vi "Insert Front Panel.vi"(8 "error in (no error)":errorcluster, 9 "Insertion Request Time":timestamp, 10 "Protected Subpanel":T1, 11 "User Manager View in":refnum<class "User Manager View.lvclass">) -> (0 "error out":errorcluster, 3 "User Manager View out":refnum<class "User Manager View.lvclass">)   [LabVIEW 2017, in "User Manager View.lvlib" / "User Manager View.lvclass"]
doc: "<License>\nCopyright © 2017 Composed Systems, LLC | All rights reserved\nwww.composed.io\n\nAuthor: Ethan Stern <ethan.stern@composed.io>\n\nThis software is provided \"AS IS\" WITHOUT WARRANTIES, either express or implied, AND IS FOR EDUCATIONAL PURPOSES ONLY.\n</License>"
uses:
  User Manager View.lvclass
  <vilib>/gpm_packages/@cs/mva-viewable/Source/IViewable/ProtectedSubpanel/Protected Subpanel Reference.ctl
  <vilib>/gpm_packages/@cs/mva-viewable/Source/IViewable/ProtectedSubpanel/ProtectedSubpanel.lvclass
  User Manager View.lvclass/User Manager View.ctl
  <vilib>/gpm_packages/@cs/mva-viewable/Source/IViewable/IViewable/IViewable.lvclass
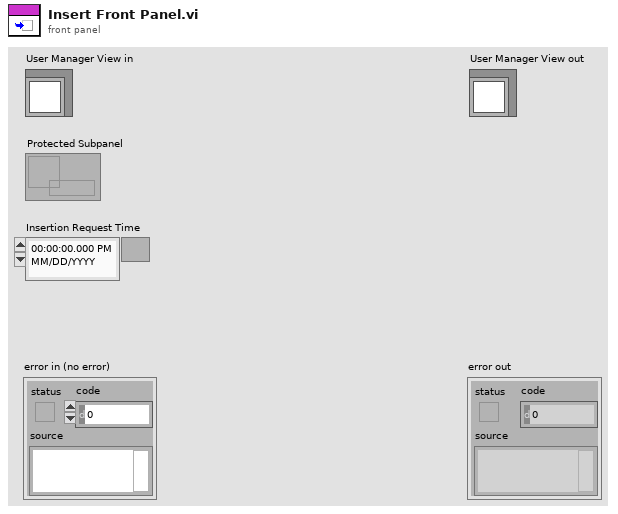
[diagram p1: front panel]
types:
  T1 = typedef "IViewable.lvlib/ProtectedSubpanel.lvclass/Protected Subpanel Reference.ctl" = refnum<data-value>
  T2 = enum8{"Enabled", "Disabled", "Disabled and Grayed Out"}
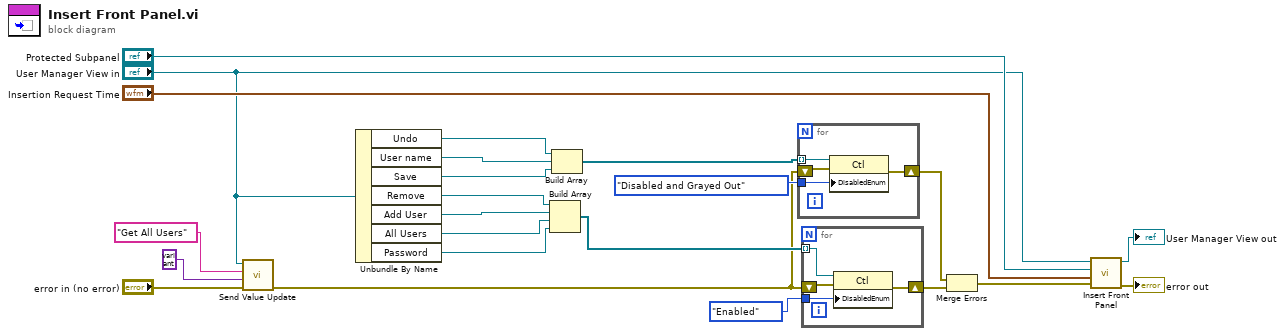
[diagram p0: block diagram]
diagram:
  n1 = call-dynamic "Send Value Update.vi"("error in (no error)"="error in (no error)", "Value"=variant, "Datum Name"="Get All Users", "IViewable in"="User Manager View in") -> ("error out"=w3:errorcluster)  [unwired: 7 in]
  n2 = Unbundle By Name("User Manager View in") -> ("Undo"=w5:refnum<vi>, "User name"=w10:refnum<vi>, "Save"=w9:refnum<vi>, "Remove"=w4:refnum<vi>, "Add User"=w15:refnum<vi>, "All Users"=w11:refnum<vi>, "Password"=w14:refnum<vi>)
  n3 = Build Array(w4, w15, w11, w14) -> (w13:refnum<vi>[])
  n4 = Build Array(w5, w10, w9) -> (w8:refnum<vi>[])
  n5 = for {
    tunnel: w8 -> [w24] mode=indexing
    tunnel: T2."Disabled and Grayed Out" ("Disabled") -> [w25]
    shift-right: [w26] -> w6
    shift-left: w3 -> [w27]
    n6 = property class="Ctl"(reference=w24, error in=w27, "DisabledEnum"=w25) -> (error out=w26:errorcluster)  [unwired: 1 out]
  }
  n7 = for {
    tunnel: w13 -> [w28] mode=indexing
    tunnel: T2."Enabled" ("Disabled") -> [w29]
    shift-right: [w30] -> w16
    shift-left: w3 -> [w31]
    n8 = property class="Ctl"(reference=w28, error in=w31, "DisabledEnum"=w29) -> (error out=w30:errorcluster)  [unwired: 1 out]
  }
  n9 = Merge Errors(w6, w16) -> (w1:errorcluster)
  n10 = call-parent "Insert Front Panel.vi"("error in (no error)"=w1, "Insertion Request Time"="Insertion Request Time", "Protected Subpanel"="Protected Subpanel", "IViewable in"="User Manager View in") -> ("error out"=→"error out":errorcluster, "IViewable out"=→"User Manager View out":refnum<class "User Manager View.lvclass">)  [unwired: 6 in]
